vi "KE622x -- Arm Init Delta Meas.vi"(0 "Resource In":refnum<visa-resource-name>, 1 "Check For SCPI Errors? (T)":bool=TRUE, 11 "error in (no error)":errorcluster) -> (4 "Resource Out (dupl)":refnum<visa-resource-name>, 15 "error out":errorcluster)   [LabVIEW 2019, in "Keithley 622x.lvlib"]
uses:
  Keithley 622x.lvlib
panel:
  in  "Init Delta Meas? (T)":bool=TRUE
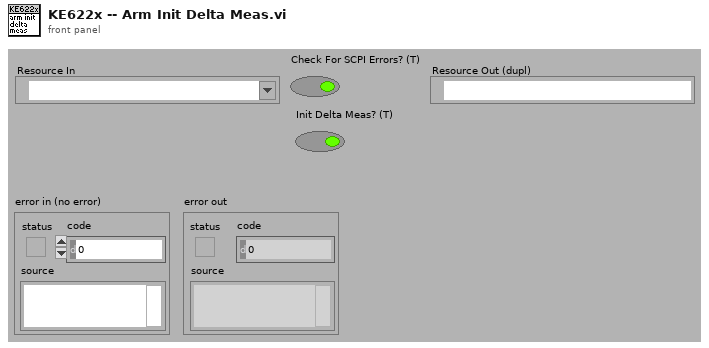
[diagram p1: front panel]
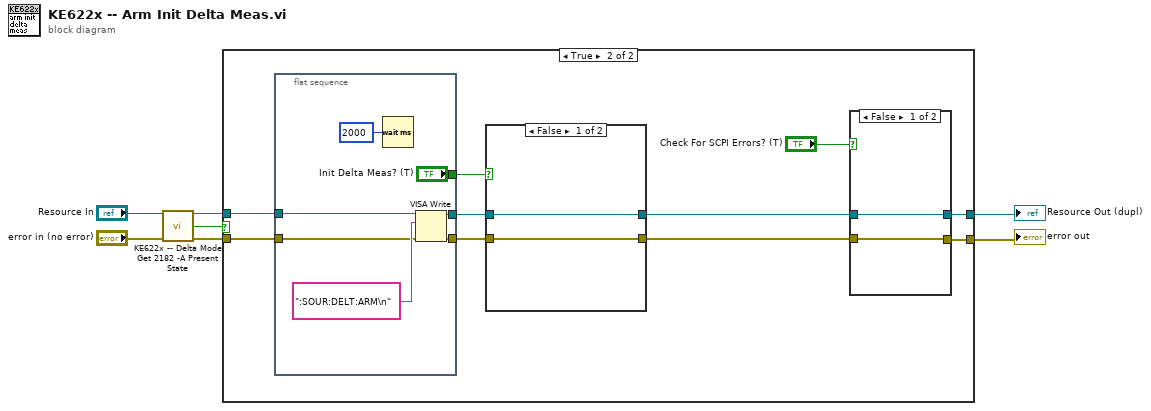
[diagram p0: block diagram]
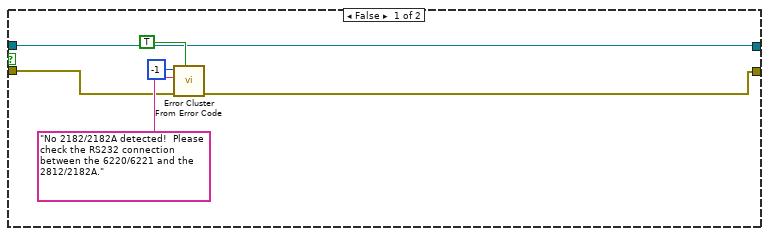
[diagram p2: hidden frame]
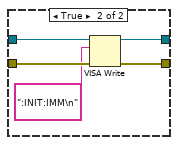
[diagram p3: hidden frame]
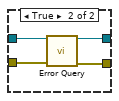
[diagram p4: hidden frame]
diagram:
  n1 = call "KE622x -- Delta Mode Get 2182 -A Present State.vi"("Resource In"="Resource In", "error in (no error)"="error in (no error)") -> ("Resource Out (dupl)"=w3:refnum<visa-resource-name>, "2182/2182A Present?"=w5:bool, "error out"=w4:errorcluster)  [unwired: 11 in]
  n2 = case shown="True" w5 {
    tunnel: w4 -> [w11 w22]
    tunnel: w3 -> [w8 w21]
    tunnel: [w8 w15] -> w2
    tunnel: [w9 w14] -> w1
    frame False {
      n3 = call <vilib>:"Error Cluster From Error Code.vi"("show call chain? (False)"=TRUE, "error in (no error)"=w11, "error message (\"\")"="No 2182/2182A detected!  Please check the RS232 connection between the 6220/6221 and the 2812/2182A.", "error code (0)"=-1) -> ("error out"=w9:errorcluster)  [unwired: 5 in]
    }
    frame True {
      n4 = flat-sequence {
        tunnel: w22 -> [w29]
        tunnel: w21 -> [w28]
        tunnel: ["Init Delta Meas? (T)"] -> w20
        tunnel: [w26] -> w19
        tunnel: [w25] -> w18
        frame #0 {
          n5 = Wait (ms)(milliseconds to wait=u32 2000) -> ()  [unwired: 1 out]
          n6 = VISA Write(VISA resource name=w28, write buffer=":SOUR:DELT:ARM\n" ("format string"), error in (no error)=w29) -> (VISA resource name out=w26:refnum<visa-resource-name>, error out=w25:errorcluster)  [unwired: 1 out]
        }
      }
      n7 = case shown="False" w20 {
        tunnel: w19 -> [w32 w37]
        tunnel: w18 -> [w31 w36]
        tunnel: [w31 w34] -> w17
        tunnel: [w32 w33] -> w16
        frame False {
        }
        frame True {
          n8 = VISA Write(VISA resource name=w37, write buffer=":INIT:IMM\n", error in (no error)=w36) -> (VISA resource name out=w33:refnum<visa-resource-name>, error out=w34:errorcluster)  [unwired: 1 out]
        }
      }
      n9 = case shown="False" "Check For SCPI Errors? (T)" {
        tunnel: w16 -> [w39 w43]
        tunnel: w17 -> [w38 w42]
        tunnel: [w38 w41] -> w14
        tunnel: [w39 w40] -> w15
        frame False {
        }
        frame True {
          n10 = call "Error Query.vi"("VISA Resource In"=w43, "error in (no error)"=w42) -> ("VISA Resource Out (dupl)"=w40:refnum<visa-resource-name>, "error out"=w41:errorcluster)  [unwired: 10 in, 2 out]
        }
      }
    }
  }
  "Resource Out (dupl)" <- w2
  "error out" <- w1
